vi "API_Start Inspecting.vi"(6 "Display Offset (in.)":dbl, 8 "error in (no error)":errorcluster, 9 "Samples Per Inch":i32, 10 "Inspect.Length (in.)":dbl, 11 "Inspect.Start (in.)":dbl) -> (0 "error out":errorcluster, 1 "ScanLength(in.)":dbl, 2 "PhysicalEndPos(in.)":dbl, 3 "PhysicalStartPos(in.)":dbl, 5 "Sample Data Notifier":refnum<notifier>)   [LabVIEW 2015, in "Tool Module.lvlib"]
doc: "Send the inspection start message to the tool manager. The Start Position and Length are checked against the tools max and min axial limits as well as the configured software limits. The actual values used are returned and can be used to set up limits needed for scan processing. \n\nThis vi also creates a notifier reference that will be used to retrieve live sample data as the inspection progresses.\n\nInput Parameters:\nStart Position (in.) The fully extended position where the (backward) scan will start.\nLength(in.) The relative length of the scan from the Start Position (must be negative).\nMax Samples Set the data collection buffer size.\n\nOutput Parameters: (These are the final values to be used after limits checking).\nPosToStartScan(in.) Scan Start position in encoder counts (this is at the extended/far end).\nPosToEndScan(in.) Scan End position in encoder counts (this is at the near end).\nScanLength(in.) Scan length to be used (after limits checking).\n\n<b>Note:</b> This VI was modified by the <b>Validate DQMH Module</b> tool to turn off automatic error handling."
uses:
  Tool Module.lvlib
  Support/_Sample Data Rtn Cluster--typedef.ctl
  Tool Config/Tool Cfg.lvlib
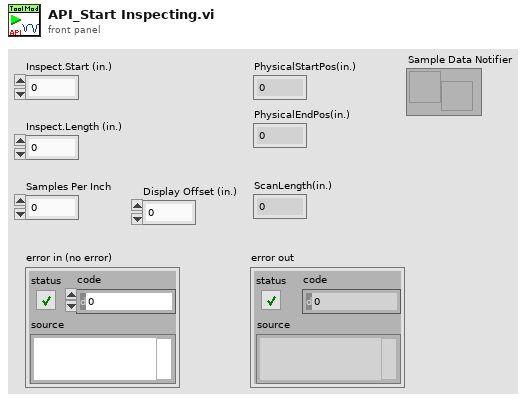
[diagram p1: front panel]
types:
  T1 = typedef "Tool Module.lvlib/INSPECT (Reply Payload)--cluster.ctl" = cluster{"Sample Data Notifier":refnum<notifier>, "INSPECT_error":errorcluster}
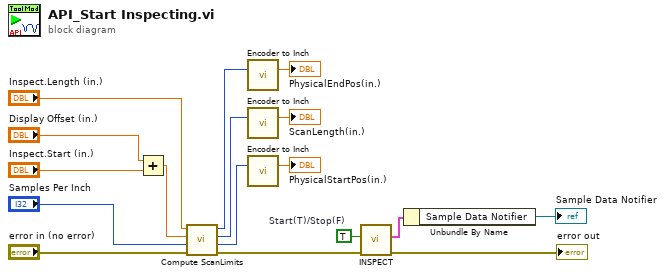
[diagram p0: block diagram]
diagram:
  w2 = TRUE  # Start(T)/Stop(F)
  n1 = Add(x="Display Offset (in.)", y="Inspect.Start (in.)") -> (x+y=w5:dbl)
  n2 = call "Compute ScanLimits.vi"("error in (no error)"="error in (no error)", "Samples Per Inch"="Samples Per Inch", "Inspect Start Axial Position"=w5, "Inspect Axial Length"="Inspect.Length (in.)") -> ("error out"=w12:errorcluster, "PosToStartScan(Cnts)"=w7:i32, "ScanLength(Cnts)"=w9:i32, "PosToEndScan(Cnts)"=w11:i32)  [unwired: 3 in, 1 out]
  n3 = call "Encoder to Inch.vi"("Encoder in"=w11) -> ("Encoder out(in)"=→"PhysicalEndPos(in.)":dbl)  [unwired: 14 in]
  n4 = call "Encoder to Inch.vi"("Encoder in"=w9) -> ("Encoder out(in)"=→"ScanLength(in.)":dbl)  [unwired: 14 in]
  n5 = call "Encoder to Inch.vi"("Encoder in"=w7) -> ("Encoder out(in)"=→"PhysicalStartPos(in.)":dbl)  [unwired: 14 in]
  n6 = call "INSPECT.vi"("error in (no error)"=w12, "Start(T)/Stop(F)"=w2) -> ("error out"=→"error out":errorcluster, "Reply Payload"=w1:T1)  [unwired: 7 in, 1 out]
  n7 = Unbundle By Name(w1) -> ("Sample Data Notifier"=→"Sample Data Notifier":refnum<notifier>)
